vi "Change UI LED Outfit.vi"(7 "State":enum16{"閒置", "進行中", "完成", "錯誤"}(ring), 8 "error in":errorcluster, 9 "Text":string, 10 "ON?":bool=TRUE, 11 "UI reference":refnum<vi>) -> (0 "error out":errorcluster)   [LabVIEW 2017, in "Toolbox.lvlib"]
uses:
  Toolbox.lvlib
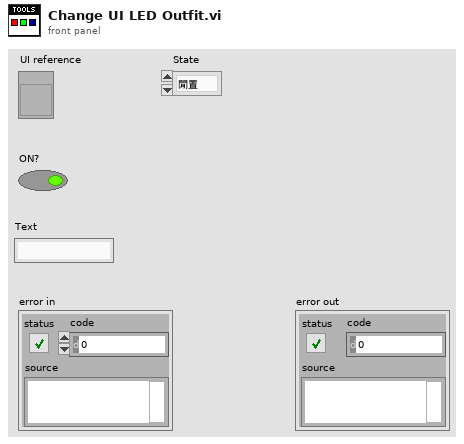
[diagram p1: front panel]
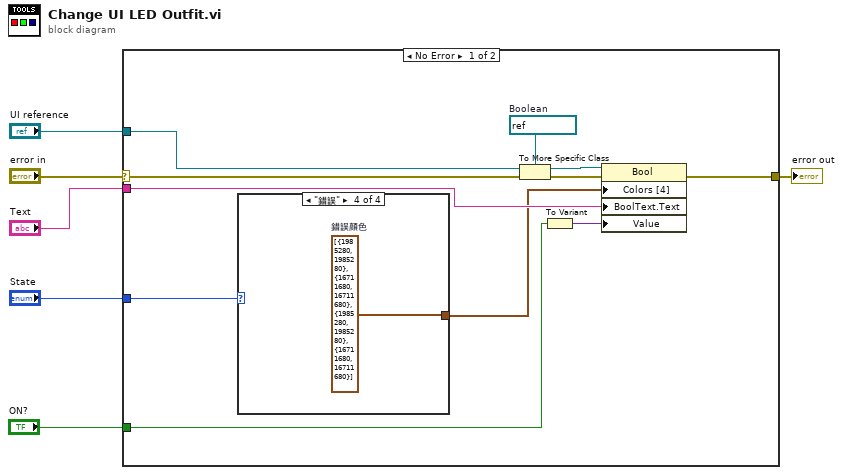
[diagram p0: block diagram]
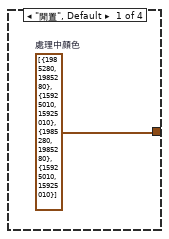
[diagram p2: hidden frame]
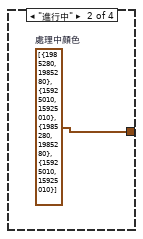
[diagram p3: hidden frame]
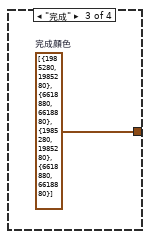
[diagram p4: hidden frame]
diagram:
  n1 = case shown="No Error" "error in" {
    selector: "error in" -> [w12 w22]
    tunnel: "UI reference" -> [w17 _]
    tunnel: "State" -> [w13 _]
    tunnel: [w11 w22] -> w1
    tunnel: "Text" -> [w10 _]
    tunnel: "ON?" -> [w8 _]
    frame No Error {
      w16 = refnum<vi> refnum  # Boolean
      n2 = case shown="\"錯誤\"" w13 {
        tunnel: [w18 w19 w20 w21] -> w7
        frame "閒置", Default {
          w18 = cluster{"Color Box":u32, "Color Box 2":u32}[] [{"Color Box"=1985280, "Color Box 2"=1985280}, {"Color Box"=15925010, "Color Box 2"=15925010}, {"Color Box"=1985280, "Color Box 2"=1985280}, {"Color Box"=15925010, "Color Box 2"=15925010}]  # 處理中顏色
        }
        frame "進行中" {
          w19 = cluster{"Color Box":u32, "Color Box 2":u32}[] [{"Color Box"=1985280, "Color Box 2"=1985280}, {"Color Box"=15925010, "Color Box 2"=15925010}, {"Color Box"=1985280, "Color Box 2"=1985280}, {"Color Box"=15925010, "Color Box 2"=15925010}]  # 處理中顏色
        }
        frame "完成" {
          w20 = cluster{"Color Box":u32, "Color Box 2":u32}[] [{"Color Box"=1985280, "Color Box 2"=1985280}, {"Color Box"=6618880, "Color Box 2"=6618880}, {"Color Box"=1985280, "Color Box 2"=1985280}, {"Color Box"=6618880, "Color Box 2"=6618880}]  # 完成顏色
        }
        frame "錯誤" {
          w21 = cluster{"Color Box":u32, "Color Box 2":u32}[] [{"Color Box"=1985280, "Color Box 2"=1985280}, {"Color Box"=16711680, "Color Box 2"=16711680}, {"Color Box"=1985280, "Color Box 2"=1985280}, {"Color Box"=16711680, "Color Box 2"=16711680}]  # 錯誤顏色
        }
      }
      n3 = To More Specific Class(target class=w16, reference=w17, error in=w12) -> (specific class reference=w15:refnum<vi>, error out=w14:errorcluster)
      n4 = To Variant(anything=w8) -> (Variant=w9:variant)
      n5 = property class="Bool"(reference=w15, error in=w14, "Colors [4]"=w7, "BoolText.Text"=w10, "Value"=w9) -> (error out=w11:errorcluster)  [unwired: 1 out]
    }
    frame Error {
    }
  }
  "error out" <- w1
